vi "manualDAQ_diag.vi"(6 "minimum value":dbl=-5.0 format="%0.2f", 7 "Rate":dbl, 8 "error in (no error)":errorcluster, 9 "Samples per Channel":i32, 10 "maximum value":dbl=5.0 format="%0.2f", 11 "physical channels":tag) -> (0 "error out":errorcluster, 3 "output waveform":waveform(dbl))   [LabVIEW 2015]
uses:
  <vilib>/DAQmx/read.llb/DAQmx Read (Analog 1D DBL 1Chan NSamp).vi
  <vilib>/DAQmx/create/channels.llb/DAQmx Create Channel (AI-Voltage-Basic).vi
  <vilib>/DAQmx/configure/timing.llb/DAQmx Timing (Sample Clock).vi
  <vilib>/DAQmx/miscellaneous.llb/DAQmx Fill In Error Info.vi
  <resource>/objmgr/daqmx.rc
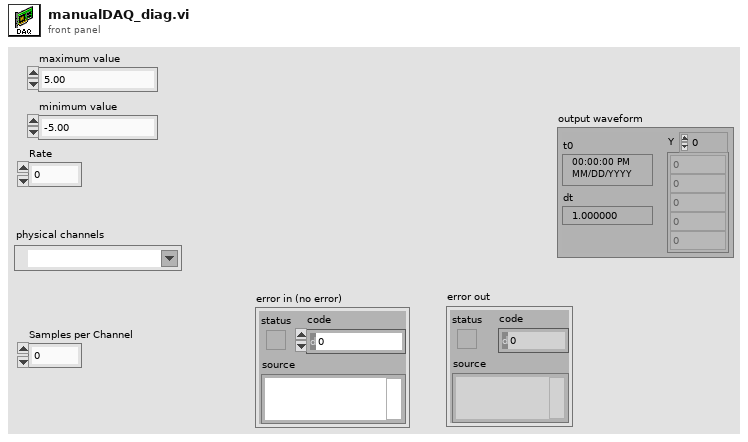
[diagram p1: front panel]
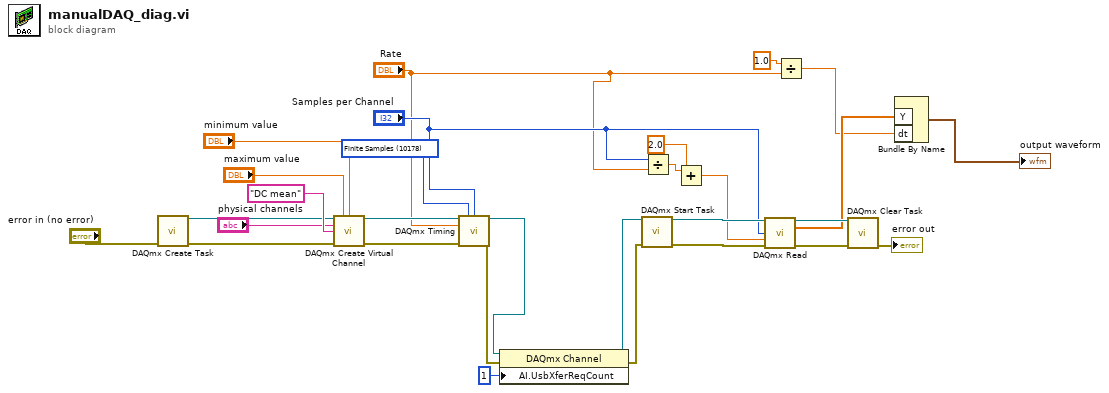
[diagram p0: block diagram]
diagram:
  w28 = 10178 items=["Finite Samples"=10178, "Continuous Samples"=10123] ("sample mode")
  n1 = call <vilib>:"DAQmx Create Task.vi"("error in"="error in (no error)") -> ("task out"=w6:refnum<k21>, "error out"=w7:errorcluster)  [unwired: 13 in]
  n2 = call-poly <vilib>:"DAQmx Create Virtual Channel.vi"("task in"=w6, "maximum value"="maximum value", "minimum value"="minimum value", "physical channels"="physical channels", "name to assign"="DC mean" ("new task name"), "error in"=w7) -> ("task out"=w17:refnum<k21>, "error out"=w18:errorcluster)  [unwired: 8 in]
  n3 = call-poly <vilib>:"DAQmx Timing.vi"("task/channels in"=w17, "sample mode"=w28, "samples per channel"="Samples per Channel", "rate"="Rate", "error in"=w18) -> ("task out"=w2:refnum<k21>, "error out"=w4:errorcluster)  [unwired: 9 in]
  n4 = property class="DAQmx Channel"(reference=w2, error in=w4, "AI.UsbXferReqCount"=u32 1) -> (reference out=w1:refnum<k21>, error out=w3:errorcluster)
  n5 = call <vilib>:"DAQmx Start Task.vi"("task/channels in"=w1, "error in"=w3) -> ("task out"=w26:refnum<k21>, "error out"=w24:errorcluster)  [unwired: 12 in]
  n6 = Divide(x="Samples per Channel", y="Rate") -> (x/y=w11:dbl)
  n7 = Add(x=w11, y=2.0) -> (x+y=w9:dbl)
  n8 = call-poly <vilib>:"DAQmx Read.vi"("task/channels in"=w26, "number of samples per channel"="Samples per Channel", "timeout"=w9, "error in"=w24) -> ("task out"=w27:refnum<k21>, "data"=w23:dbl[], "error out"=w29:errorcluster)  [unwired: 9 in]
  n9 = Divide(x=1.0, y="Rate") -> (x/y=w21:dbl)
  n10 = call <vilib>:"DAQmx Clear Task.vi"("task in"=w27, "error in"=w29) -> ("error out"=→"error out":errorcluster)  [unwired: 13 in]
  n11 = Bundle By Name("Y"=w23, "dt"=w21) -> (→"output waveform":waveform(dbl))  [unwired: 1 in]
